vi "Test Top Level.vi"() -> ()   [LabVIEW 2011]
panel:
  in  "Case Constant\n(See Context Help)":bool
  in  "OK":bool
  out "Message":string
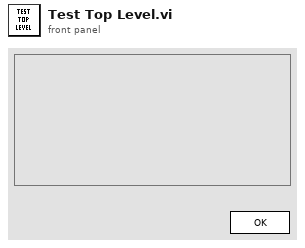
[diagram p1: front panel]
types:
  T1 = cluster{"left":i16, "top":i16, "right":i16, "bottom":i16}
  T2 = enum32{"invalid app kind", "Development System", "Run Time System", "Student Edition", "Embedded LabVIEW", "Evaluation", "Custom"}
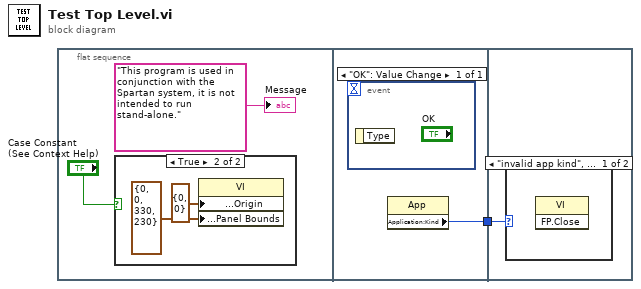
[diagram p0: block diagram]
diagram:
  n1 = flat-sequence {
    tunnel: [w6] -> w1
    tunnel: w1 -> [w7]
    frame #0 {
      n2 = case shown="True" "Case Constant\n(See Context Help)" {
        frame False {
        }
        frame True {
          n3 = property class="VI"("Front Panel Window:Origin"=cluster{"Horizontal":i16, "Vertical":i16} {"Horizontal"=0, "Vertical"=0}, "Front Panel Window:Panel Bounds"=T1 {"left"=0, "top"=0, "right"=330, "bottom"=230}) -> ()  [unwired: 2 in, 2 out]
        }
      }
      "Message" <- "This program is used in conjunction with the Spartan system, it is not intended to run stand-alone."
    }
    frame #1 {
      n4 = event shown="[0] \"OK\": Value Change" {
        selector: _ -> [_]
        dyn-events: _ -> [_]
        timeout: _ -> [_]
        event "OK": Value Change {
          n5 = event-data() -> ()  [unwired: 2 out]
        }
      }
      n6 = property class="App"() -> ("Application:Kind"=w6:T2)  [unwired: 2 in, 2 out]
    }
    frame #2 {
      n7 = case shown="\"invalid app kind\", Default" w7 {
        frame "invalid app kind", Default {
          n8 = invoke class="VI" method="FP.Close"() -> ()  [unwired: 3 in, 3 out]
        }
        frame "Development System" {
        }
      }
    }
  }
